vi "File.Add Name Suffix.vi"(9 "Suffix":string, 11 "Source":path) -> (0 "error out":errorcluster, 3 "New Path":path)   [LabVIEW 2024]
uses:
  File Utils.lvlib
panel:
  out "Dir":bool
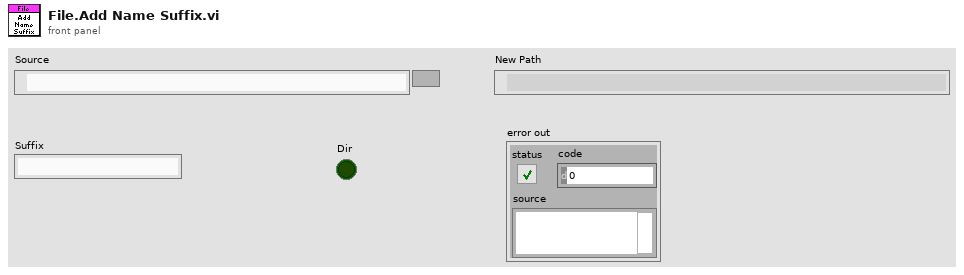
[diagram p1: front panel]
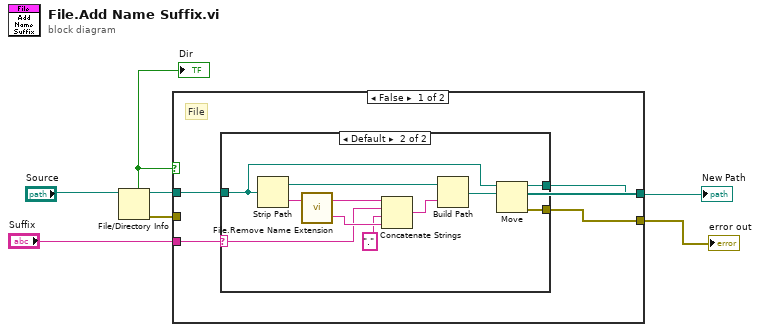
[diagram p0: block diagram]
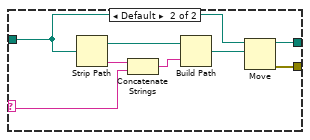
[diagram p4: hidden frame]
diagram:
  n1 = File/Directory Info(path="Source") -> (path out=w7:path, directory=w6:bool, error out=w5:errorcluster)  [unwired: 1 in, 4 out]
  "Dir" <- w6
  n2 = case shown="False" w6 {
    tunnel: [w9 w25] -> w2
    tunnel: w7 -> [w11 w27]
    tunnel: w5 -> [_ _]
    tunnel: "Suffix" -> [w8 w24]
    tunnel: [w10 w26] -> w1
    frame False {
      # "File"
      n3 = case shown="Default" w8 {
        selector: w8 -> [_ w13]
        tunnel: w11 -> [w12 w16]
        tunnel: [_ w15] -> w10
        tunnel: [w12 w14] -> w9
        frame "" {
        }
        frame Default {
          n4 = Strip Path(path=w16) -> (stripped path=w21:path, name=w23:string)
          n5 = call "File.Remove Name Extension.vi"("File Name"=w23) -> ("Ext"=w19:string, "Name Less Ext"=w20:string)  [unwired: 1 in]
          n6 = Concatenate Strings(w20, w13, ".", w19) -> (w22:string)
          n7 = Build Path(base path=w21, name or relative path=w22) -> (appended path=w17:path)
          n8 = Move(source path=w16, 10:w17) -> (error out=w15:errorcluster, 3:w14:path)  [unwired: 3 in, 1 out]
        }
      }
    }
    frame True {
      n9 = case shown="\"\"" w24 {
        selector: w24 -> [_ w29]
        tunnel: w27 -> [w28 w33]
        tunnel: [_ w31] -> w26
        tunnel: [w28 w30] -> w25
        frame "" {
        }
        frame Default {
          n10 = Strip Path(path=w33) -> (stripped path=w34:path, name=w36:string)
          n11 = Concatenate Strings(w36, w29) -> (w35:string)
          n12 = Build Path(base path=w34, name or relative path=w35) -> (appended path=w32:path)
          n13 = Move(source path=w33, 10:w32) -> (error out=w31:errorcluster, 3:w30:path)  [unwired: 3 in, 1 out]
        }
      }
    }
  }
  "New Path" <- w2
  "error out" <- w1
